vi "TestDynamixelExploration.vi"() -> ()   [LabVIEW 2013]
uses:
  <instrlib>/Dynamixel Motor/Dynamixel Motor.lvlib
panel:
  in  "stop":bool
  in  "Goal Position (150 deg)":dbl=150.0
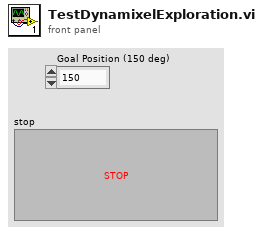
[diagram p1: front panel]
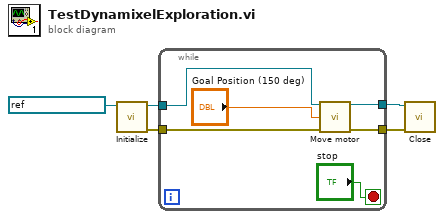
[diagram p0: block diagram]
diagram:
  n1 = call <instrlib>:"Initialize.vi"("VISA resource name"=refnum<visa-resource-name> "ASRL2::INSTR") -> ("error out"=w4:errorcluster, "VISA resource name out"=w5:refnum<visa-resource-name>)  [unwired: 9 in]
  n2 = while {
    tunnel: w5 -> [w11]
    tunnel: w4 -> [w10]
    tunnel: [w8] -> w2
    tunnel: [w7] -> w1
    stop <- "stop" stop-if-true
    n3 = call <instrlib>:"Move motor.vi"("VISA resource name"=w11, "Goal Position (150 deg)"="Goal Position (150 deg)", "error in (no error)"=w10) -> ("VISA resource name out"=w8:refnum<visa-resource-name>, "error out"=w7:errorcluster)  [unwired: 11 in]
  }
  n4 = call <instrlib>:"Close.vi"("error in (no error)"=w1, "VISA resource name"=w2) -> ()  [unwired: 9 in, 1 out]
